vi "_testNewFile.vi"() -> ()   [LabVIEW 2020]
uses:
  Source/Libraries/Ballard_Parameter_ni/_tyedefs/label_type.ctl
  Source/Libraries/Ballard_Parameter_ni/_tyedefs/parameter_type.ctl
  Source/Libraries/Ballard_Parameter_ni/Ballard_Parameter_ni.lvlib
panel:
  in  "parameter configuration":T1
  in  "label configuration":T2 {"sdi" items=["All", "Item00", "Item01", "Item10", "Item11"]}
  in  "hardwareChannel":i32
  in  "direction":i32(ring) items=["incoming", "outgoing"]
  out "error out":errorcluster
  out "SerializeXML":bool
  in  "XML path":path
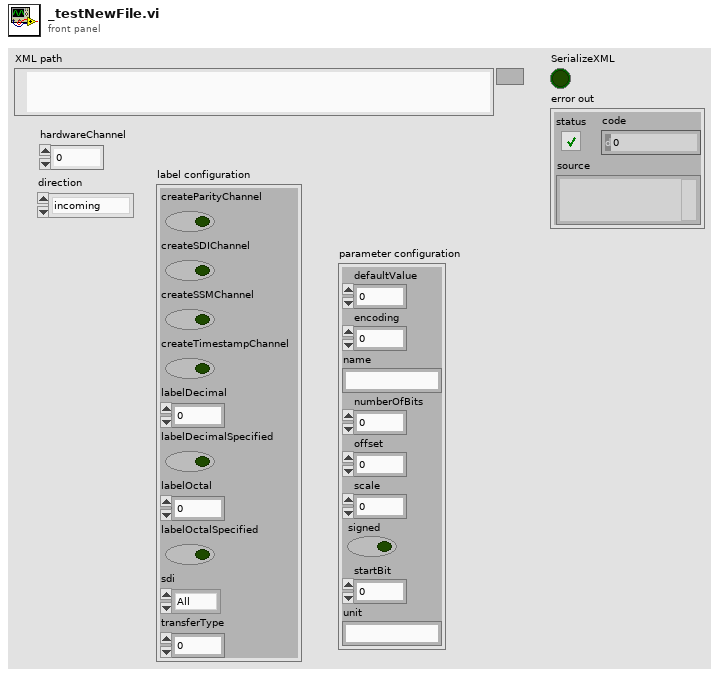
[diagram p1: front panel]
types:
  T1 = typedef "parameter_type.ctl" = cluster{"defaultValue":dbl, "encoding":i32, "name":string, "numberOfBits":i32, "offset":dbl, "scale":dbl, "signed":bool, "startBit":i32, "unit":string}
  T2 = typedef "label_type.ctl" = cluster{"createParityChannel":bool, "createSDIChannel":bool, "createSSMChannel":bool, "createTimestampChannel":bool, "labelDecimal":i32, "labelDecimalSpecified":bool, "labelOctal":i32, "labelOctalSpecified":bool, "sdi":i32, "transferType":i32}
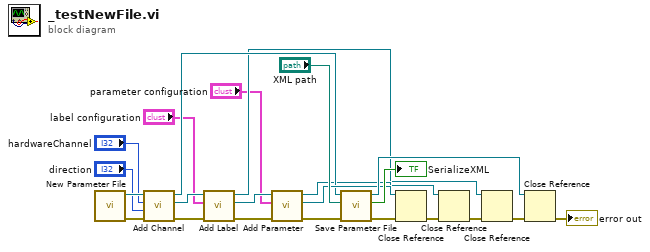
[diagram p0: block diagram]
diagram:
  n1 = call "New Parameter File.vi"() -> ("error out"=w19:errorcluster, "new parameter file"=w18:refnum<k24>)  [unwired: 10 in]
  n2 = call "Add Channel.vi"("error in"=w19, "direction"="direction", "hardwareChannel"="hardwareChannel", "parameter file in"=w18) -> ("error out"=w15:errorcluster, "new channel"=w17:refnum<k24>, "parameter file out"=w14:refnum<k24>)  [unwired: 5 in]
  n3 = call "Add Label.vi"("error in"=w15, "label configuration"="label configuration", "channel in"=w17) -> ("error out"=w11:errorcluster, "new label"=w12:refnum<k24>, "channel out"=w9:refnum<k24>)  [unwired: 6 in]
  n4 = call "Add Parameter.vi"("error in"=w11, "parameter configuration"="parameter configuration", "label in"=w12) -> ("error out"=w3:errorcluster, "new parameter"=w16:refnum<k24>, "label out"=w10:refnum<k24>)  [unwired: 6 in]
  n5 = call "Save Parameter File.vi"("error in"=w3, "XML path"="XML path", "parameter file in"=w14) -> ("error out"=w2:errorcluster, "SerializeXML"=→"SerializeXML":bool, "parameter file out"=w23:refnum<k24>)  [unwired: 6 in]
  n6 = Close Reference(reference=w16, error in (no error)=w2) -> (error out=w13:errorcluster)
  n7 = Close Reference(reference=w10, error in (no error)=w13) -> (error out=w8:errorcluster)
  n8 = Close Reference(reference=w9, error in (no error)=w8) -> (error out=w1:errorcluster)
  n9 = Close Reference(reference=w23, error in (no error)=w1) -> (error out=→"error out":errorcluster)
